vi "Set Editor Position.vi"(8 "error in":errorcluster, 11 "Editor Ref":refnum<vi>) -> (0 "error out":errorcluster)   [LabVIEW 2021, in "lv_icon.lvlib"]
doc: "Reads the position from the LabVIEW INI file and sets the position of the editor. If the INI token is missing or formatted incorrectly, the editor will be centered on the caller's monitor."
uses:
  <vilib>/LabVIEW Icon API/lv_icon/lv_icon.lvlib
  <vilib>/Utility/miscctls.llb/LVRectTypeDef.ctl
  <resource>/dialog/lvconfig.llb/LV Config Read Boolean.vi
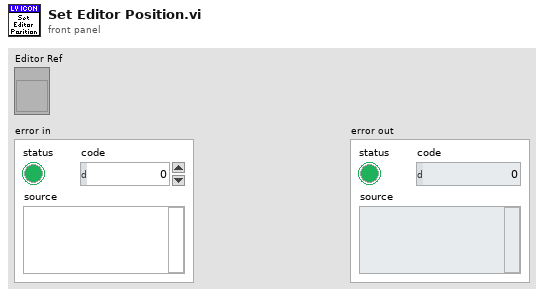
[diagram p1: front panel]
types:
  T1 = typedef "LVRectTypeDef.ctl" = cluster{"Left":i16, "Top":i16, "Right":i16, "Bottom":i16}
  T2 = typedef "LVAllMonitorsDisplayTypeDef.ctl" = cluster{"Bounds":cluster{"Left":i16, "Top":i16, "Right":i16, "Bottom":i16}, "Depth":i16}[]
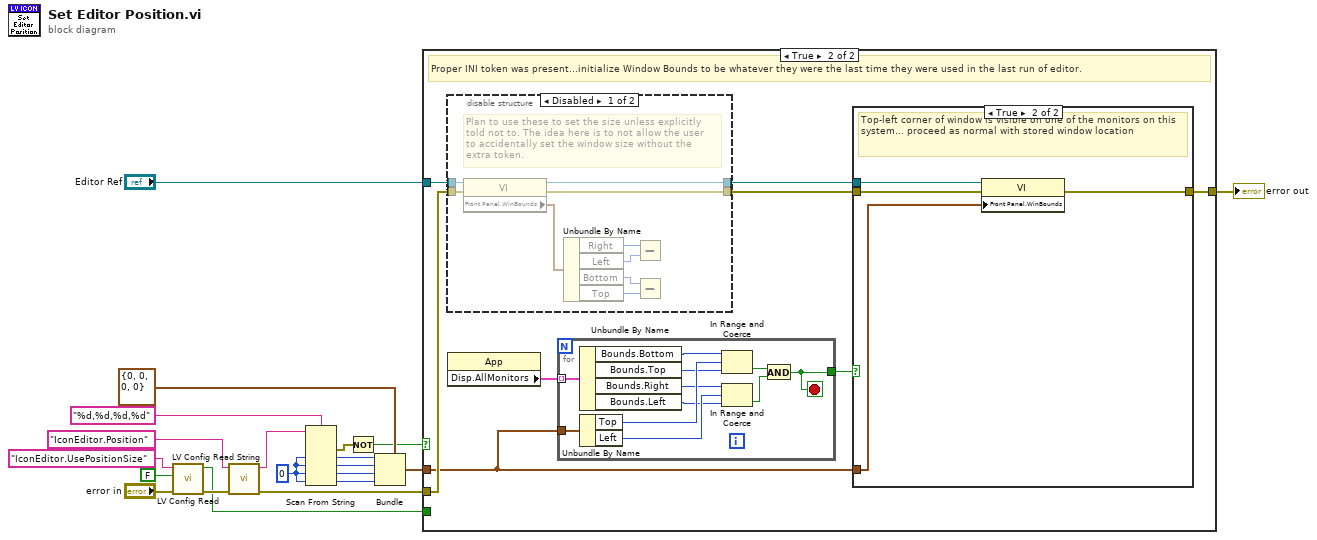
[diagram p0: block diagram]
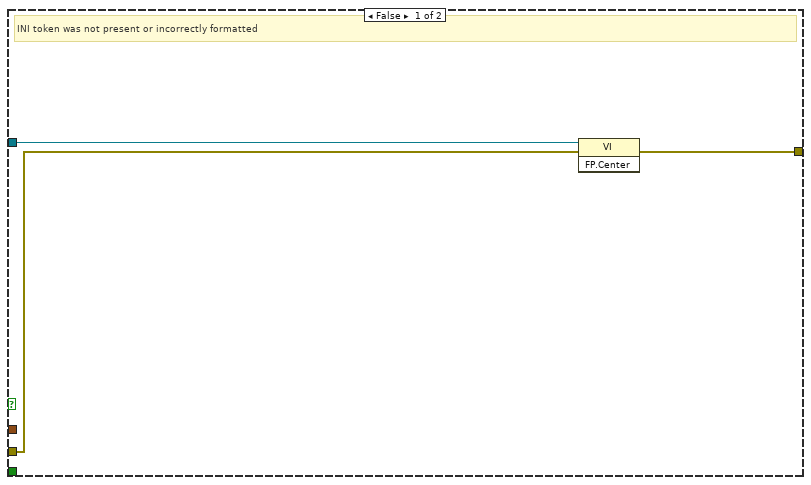
[diagram p2: hidden frame]
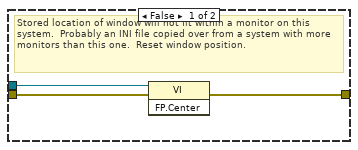
[diagram p4: hidden frame]
diagram:
  w4 = i16 0 ("default value 1")
  n1 = call-poly <resource>:"LV Config Read.vi"("error in"="error in", "default value"=FALSE, "key"="IconEditor.UsePositionSize") -> ("error out"=w18:errorcluster, "value"=w14:bool)  [unwired: 2 in, 1 out]
  n2 = call <resource>:"LV Config Read String.vi"("error in"=w18, "key"="IconEditor.Position") -> ("error out"=w17:errorcluster, "value"=w2:string)  [unwired: 3 in, 1 out]
  n3 = Scan From String(format string="%d,%d,%d,%d", input string=w2, default 1=w4, default 2=w4, default 3=w4, default 4=w4) -> (error out=w16:errorcluster, output 1=w7:i16, output 2=w8:i16, output 3=w9:i16, output 4=w10:i16)  [unwired: 2 in, 2 out]
  n4 = Not(x=w16) -> (.not. x?=w1:bool)
  n5 = Bundle(cluster=T1 {"Left"=0, "Top"=0, "Right"=0, "Bottom"=0} ("Front Panel Window:Window Bounds"), "Left"=w7, "Top"=w8, "Right"=w9, "Bottom"=w10) -> (w3:T1)
  n6 = case shown="True" w1 {
    tunnel: w14 -> [_ _]
    tunnel: "Editor Ref" -> [w21 w26]
    tunnel: [w23 w31] -> w20
    tunnel: w17 -> [w22 w29]
    tunnel: w3 -> [_ w24]
    frame False {
      # "INI token was not present or incorrectly formatted"
      n7 = invoke class="VI" method="FP.Center"(reference=w21, error in=w22) -> (error out=w23:errorcluster)  [unwired: 1 in, 2 out]
    }
    frame True {
      # "Proper INI token was present...initialize Window Bounds to be whatever they were the last time they were used in the last run of editor."
      n8 = disable-structure shown="Disabled" {
        disable-tunnel: w26 -> [w38 w41]
        disable-tunnel: w29 -> [w40 w42]
        disable-tunnel: [w32 w41] -> w25
        disable-tunnel: [w39 w42] -> w30
        frame Disabled {
          # "Plan to use these to set the size unless explicitly\ntold not to. The idea here is to not allow the user\nto accidentally set the window size without the\nextra token."
          n9 = property class="VI"(reference=w38, error in=w40) -> (reference out=w32:refnum<vi>, error out=w39:errorcluster, "Front Panel.WinBounds"=w37:T1)
          n10 = Unbundle By Name(w37) -> ("Right"=w36:i16, "Left"=w35:i16, "Bottom"=w34:i16, "Top"=w33:i16)
          n11 = Subtract(x=w36, y=w35) -> ()  [unwired: 1 out]
          n12 = Subtract(x=w34, y=w33) -> ()  [unwired: 1 out]
        }
        frame Enabled {
        }
      }
      n13 = property class="App"() -> ("Disp.AllMonitors"=w28:T2)  [unwired: 2 in, 2 out]
      n14 = for {
        tunnel: w28 -> [w58] mode=indexing
        tunnel: [w51] -> w27
        tunnel: w24 -> [w50]
        stop <- w51 stop-if-true
        n15 = Unbundle By Name(w58) -> ("Bounds.Bottom"=w54:i16, "Bounds.Top"=w55:i16, "Bounds.Right"=w57:i16, "Bounds.Left"=w56:i16)
        n16 = Unbundle By Name(w50) -> ("Top"=w59:i16, "Left"=w60:i16)
        n17 = In Range and Coerce(upper limit=w54, x=w59, lower limit=w55) -> (In Range?=w53:bool)  [unwired: 1 out]
        n18 = In Range and Coerce(upper limit=w57, x=w60, lower limit=w56) -> (In Range?=w52:bool)  [unwired: 1 out]
        n19 = And(x=w53, y=w52) -> (x .and. y?=w51:bool)
      }
      n20 = case shown="True" w27 {
        tunnel: w24 -> [_ w47]
        tunnel: w25 -> [w43 w46]
        tunnel: w30 -> [w45 w49]
        tunnel: [w44 w48] -> w31
        frame False {
          # "Stored location of window will not fit within a monitor on this system.  Probably an INI file copied over from a system with more monitors than this one.  Reset window position."
          n21 = invoke class="VI" method="FP.Center"(reference=w43, error in=w45) -> (error out=w44:errorcluster)  [unwired: 1 in, 2 out]
        }
        frame True {
          # "Top-left corner of window is visible on one of the monitors on this system... proceed as normal with stored window location"
          n22 = property class="VI"(reference=w46, error in=w49, "Front Panel.WinBounds"=w47) -> (error out=w48:errorcluster)  [unwired: 1 out]
        }
      }
    }
  }
  "error out" <- w20
